vi "Execute-Endurance-Test.vi"   [LabVIEW 2014]
uses:
  <vilib>/Utility/error.llb/DialogType.ctl
  <vilib>/Wiresmith Technology/LabVIEW CLI/CLI Class/CLI.lvclass
types:
  T1 = typedef "DialogType.ctl" = u16
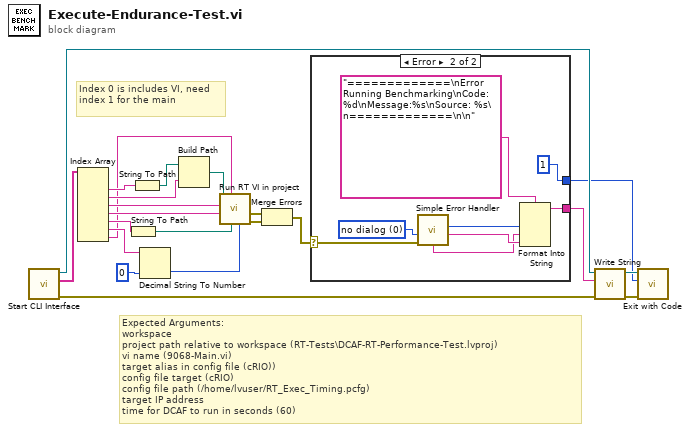
[diagram p0: block diagram]
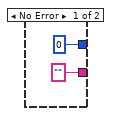
[diagram p2: hidden frame]
diagram:
  # "Index 0 is includes VI, need index 1 for the main"
  # "Expected Arguments:\nworkspace \nproject path relative to workspace (RT-Tests\\DCAF-RT-Performance-Test.lvproj)\nvi name (9068-Main.vi)\ntarget alias in config file (cRIO))\nconfig file target (cRIO)\nconfig file path (/home/lvuser/RT_Exec_Timing.pcfg)\ntarget IP address\ntime for DCAF to run in seconds (60)"
  n1 = call <vilib>:"Start CLI Interface.vi"() -> ("error out"=w16:errorcluster, "Custom Parameters"=w22:string[], "CLI out"=w18:refnum<class "CLI.lvclass">)  [unwired: 9 in]
  n2 = Index Array(array=w22) -> (element #1=w2:string, element #2=w11:string, element #3=w9:string, element #4=w8:string, element #5=w13:string, element #6=w14:string, element #7=w1:string)  [unwired: 7 in]
  n3 = String To Path(string=w13) -> (path=w7:path)
  n4 = String To Path(string=w2) -> (path=w12:path)
  n5 = Decimal String To Number(string=w14, default (0L)=u32 0 ("default (0 I32)")) -> (number=w6:u32)  [unwired: 1 in, 1 out]
  n6 = Build Path(base path=w12, name or relative path=w11) -> (appended path=w10:path)
  n7 = call "Run RT VI in project.vi"("Run Time"=w6, "configuration file path"=w7, "ip address"=w1, "target alias"=w8, "vi name"=w9, "Project Path"=w10) -> ("error out"=w5:errorcluster, "invoked VI error out"=w4:errorcluster)  [unwired: 4 in]
  n8 = Merge Errors(w4, w5) -> (w3:errorcluster)
  n9 = case shown="Error" w3 {
    selector: w3 -> [_ w29]
    tunnel: ["" w25] -> w19
    tunnel: [0 ("Exit Code (0)") 1 ("Exit Code (0)")] -> w17
    frame No Error {
    }
    frame Error {
      w30 = T1 0 items=["no dialog", "OK message", "continue or stop message", "OK message + warnings", "continue/stop + warnings"] ("type of dialog (OK msg:1)")
      n10 = call <vilib>:"Simple Error Handler.vi"("type of dialog (OK msg:1)"=w30, "error in (no error)"=w29) -> ("code out"=w28:i32, "source out"=w27:string, "message"=w26:string)  [unwired: 3 in, 2 out]
      n11 = Format Into String(format string="=============\nError Running Benchmarking\nCode: %d\nMessage:%s\nSource: %s\n=============\n\n", w28, w26, w27) -> (resulting string=w25:string)  [unwired: 2 in, 1 out]
    }
  }
  n12 = call <vilib>:"Write String.vi"("error in (no error)"=w16, "Text to Write"=w19, "CLI in"=w18) -> ("error out"=w21:errorcluster, "CLI out"=w20:refnum<class "CLI.lvclass">)  [unwired: 7 in]
  n13 = call <vilib>:"Exit with Code.vi"("error in (no error)"=w21, "Exit Code (0)"=w17, "CLI in"=w20) -> ()  [unwired: 8 in, 1 out]
